vi "Begin.vi"(11 "Image Size":T1=enum."160x120") -> (0 "error out":errorcluster)   [LabVIEW 2012]
doc: "Called before other user functions, this VI is expected to open initial I/O refnums, load in file data, and do all program initialization. Notice that the <B>error out</B> terminal is simply used for data flow. Wiring it to other structures or subVIs ensures that this VI runs first."
uses:
  <vilib>/Rock Robotics/WPI/Camera/WPI_CameraImageSize.ctl
  <vilib>/Rock Robotics/WPI/Camera/WPI_CameraWhite Balance Values.ctl
  <vilib>/Rock Robotics/WPI/Camera/WPI_CameraExposure Values.ctl
  <vilib>/Rock Robotics/WPI/Camera/WPI_CameraFrameRate.ctl
  <vilib>/Rock Robotics/SystemInterfaces/DIO/FPGA_DIOPWMChannel.ctl
  <vilib>/Rock Robotics/SystemInterfaces/Typedef/FPGA_TypedefDigitalModule.ctl
  <vilib>/Rock Robotics/SystemInterfaces/DIO/FPGA_DIOChannel.ctl
  <vilib>/Rock Robotics/WPI/Encoder/WPI_EncoderType.ctl
  <vilib>/Rock Robotics/SystemInterfaces/Typedef/FPGA_TypedefAnalogModuleForGyro.ctl
  <vilib>/Rock Robotics/SystemInterfaces/AI/FPGA_AIGyroChannel.ctl
  <vilib>/Rock Robotics/WPI/SafetyOutput/WPI_SafetyOutputConfigMenu.ctl
  <vilib>/Rock Robotics/WPI/Joystick/WPI_JoystickDeviceEnum.ctl
  <vilib>/Rock Robotics/SystemInterfaces/DIO/FPGA_DIORelayChannel.ctl
  <vilib>/Rock Robotics/SystemInterfaces/Typedef/FPGA_TypedefSolenoidModule.ctl
  <vilib>/Rock Robotics/WPI/Solenoid/WPI_SolenoidChannel.ctl
  <vilib>/Rock Robotics/WPI/MotorControl/WPI_MotorControlOpen Victor.vi
  <vilib>/Rock Robotics/WPI/Counter/WPI_CounterDigitalInputToDigitalSource.vi
  <vilib>/Rock Robotics/WPI/RobotDrive/WPI_RobotDriveOpen4MotorWithVictor.vi
  System Set Points and States.vi
  <vilib>/Rock Robotics/WPI/Counter/WPI_CounterOpen UpDown Mode.vi
  <vilib>/Rock Robotics/WPI/Solenoid/WPI_SolenoidOpenSingle.vi
  <vilib>/Rock Robotics/WPI/Compressor/WPI_CompressorGetSetRefNum.vi
panel:
  in  "Image Size 2":T1=enum."160x120"
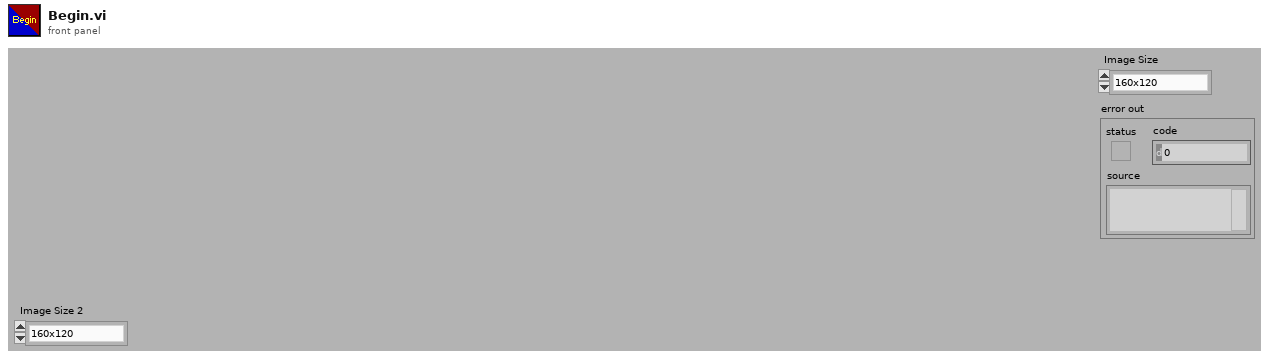
[diagram p1: front panel]
types:
  T1 = typedef "WPI_CameraImageSize.ctl" = enum16{"640x480", "320x240", "160x120"}
  T2 = typedef "WPI_SolenoidChannel.ctl" = enum8{"Solenoid 1", "Solenoid 2", "Solenoid 3", "Solenoid 4", "Solenoid 5", "Solenoid 6", "Solenoid 7", "Solenoid 8", "Invalid"}
  T3 = typedef "FPGA_TypedefSolenoidModule.ctl" = enum16{"Solenoid Module 1", "Solenoid Module 2"}
  T4 = typedef "FPGA_DIORelayChannel.ctl" = enum8{"Relay 1", "Relay 2", "Relay 3", "Relay 4", "Relay 5", "Relay 6", "Relay 7", "Relay 8", "Invalid"}
  T5 = typedef "FPGA_TypedefDigitalModule.ctl" = enum16{"Digital Module 1", "Digital Module 2"}
  T6 = typedef "FPGA_DIOChannel.ctl" = enum8{"DIO 1", "DIO 2", "DIO 3", "DIO 4", "DIO 5", "DIO 6", "DIO 7", "DIO 8", "DIO 9", "DIO 10", "DIO 11", "DIO 12", "DIO 13", "DIO 14", "Invalid"}
  T7 = typedef "WPI_EncoderType.ctl" = enum16{"1x", "2x", "4x"}
  T8 = typedef "WPI_JoystickDeviceEnum.ctl" = enum16{"USB 1", "USB 2", "USB 3", "USB 4", "Kinect 1", "Kinect 2"}
  T9 = typedef "WPI_CameraFrameRate.ctl" = u32
  T10 = typedef "WPI_CameraExposure Values.ctl" = enum16{"Auto", "Flicker-free 50 Hz", "Flicker-free 60 Hz", "Hold current"}
  T11 = typedef "WPI_CameraWhite Balance Values.ctl" = enum16{"Auto", "Fixed indoor", "Fixed outdoor 1", "Fixed outdoor 2", "Fixed fluorescent 1", "Fixed fluorescent 2", "Hold current"}
  T12 = typedef "WPI_SafetyOutputConfigMenu.ctl" = enum16{"Enable", "Disable"}
  T13 = typedef "FPGA_AIGyroChannel.ctl" = enum8{"AI 1", "AI 2", "Invalid"}
  T14 = typedef "FPGA_TypedefAnalogModuleForGyro.ctl" = enum16{"Analog Module 1"}
  T15 = typedef "FPGA_DIOPWMChannel.ctl" = enum8{"PWM 1", "PWM 2", "PWM 3", "PWM 4", "PWM 5", "PWM 6", "PWM 7", "PWM 8", "PWM 9", "PWM 10", "Invalid"}
  T16 = typedef "WPI_RobotDriveDevRef.ctl" = cluster{"DevStatus":errorcluster, "Motors[]":T17[], "Square Inputs":bool, "Max Output":dbl, "Isochronous":bool}
  T17 = typedef "WPI_MotorControlDeviceRef.ctl" = cluster{"DeviceStatus":errorcluster, "Type":enum16{"PWM", "CAN"}, "PWM":cluster{"Digital Module":T5, "PWM Channel":T15, "DeadBand":T18}, "CAN":cluster{"Device Number":u8, "Control Mode":T19, "Semaphore":T20, "Max Vout":dbl}, "Invert":bool, "TransformRef":T21, "InvTransformRef":T21}
  T18 = typedef "WPI_PWMDeadband.ctl" = cluster{"Name":string, "maxPositivePwm":i32, "minPositivePwm":i32, "centerPwm":i32, "maxNegativePwm":i32, "minNegativePwm":i32, "angularRange":u16}
  T19 = typedef "WPI_CANJaguar_ControlMode.ctl" = enum8{"Percent VBus", "Current", "Speed", "Position", "Voltage"}
  T20 = typedef "Semaphore RefNum" = refnum<k1>
  T21 = typedef "WPI_PWMTransform_ConPane.ctl" = refnum<vi>
  T22 = typedef "WPI_CameraDevRef.ctl" = cluster{"Camera Address":string, "CameraStatus":errorcluster, "Acquire Image Notifier":refnum<notifier>}
  T23 = typedef "WPI_DigitalInputDevRef.ctl" = cluster{"DevStatus":errorcluster, "DIO Channel":T6, "Digital Module":T5}
  T24 = typedef "FPGA_CounterEncoderSourceConvertionLVSourceType.ctl" = cluster{"DevStatus":errorcluster, "AnalogTriggerMode?":bool, "DigitalMode":cluster{"Digital Module":T5, "DIO Channel":T25}, "AnalogTriggerMode":cluster{"AnalogTriggerIndex":T26, "OutputType":T27}}
  T25 = typedef "FPGA_DIODigitalSourceChannel.ctl" = enum8{"DIO 1", "DIO 2", "DIO 3", "DIO 4", "DIO 5", "DIO 6", "DIO 7", "DIO 8", "DIO 9", "DIO 10", "DIO 11", "DIO 12", "DIO 13", "DIO 14", "Disabled"}
  T26 = typedef "FPGA_AnalogTriggerIndex.ctl" = enum8{"Trig 0", "Trig 1", "Trig 2", "Trig 3", "Trig 4", "Trig 5", "Trig 6", "Trig 7", "Invalid"}
  T27 = typedef "FPGA_AnalogTriggerOutType.ctl" = enum16{"InWindow", "TriggerState", "Rising", "Falling"}
  T28 = typedef "WPI_GyroDevRef.ctl" = cluster{"DevStatus":errorcluster, "Analog Module":T29, "Analog Channel":T30, "Offset":dbl, "Gain (VoltsPerDegree/Second)":dbl}
  T29 = typedef "FPGA_TypedefAnalogModule.ctl" = enum16{"Analog Module 1", "Analog Module 2"}
  T30 = typedef "FPGA_AIChannel.ctl" = enum8{"AI 1", "AI 2", "AI 3", "AI 4", "AI 5", "AI 6", "AI 7", "AI 8", "Invalid"}
  T31 = typedef "WPI_CounterDevRef.ctl" = cluster{"DevStatus":errorcluster, "CntIndex":T32}
  T32 = typedef "FPGA_CounterCtrSystemIndex.ctl" = enum8{"Ctr 0", "Ctr 1", "Ctr 2", "Ctr 3", "Ctr 4", "Ctr 5", "Ctr 6", "Ctr 7", "Invalid"}
  T33 = typedef "WPI_EncoderDevRef.ctl" = cluster{"DevStatus":errorcluster, "EncoderIndex":T34, "CounterIndex":T32, "DistancePerCount":dbl, "Decoding Type":T7}
  T34 = typedef "FPGA_EncoderIdx.ctl" = enum8{"Enc 0", "Enc 1", "Enc 2", "Enc 3", "Invalid"}
  T35 = typedef "WPI_SolenoidDevRef.ctl" = cluster{"DevStatus":errorcluster, "Solenoid Module":T3, "Forward Solenoid Channel":T2, "Reverse Solenoid Channel":T2}
  T36 = typedef "WPI_CompressorDevRef.ctl" = cluster{"DevStatus":errorcluster, "DigitalInputDevRef":T23, "RelayDevRef":T37}
  T37 = typedef "WPI_RelayDevRef.ctl" = cluster{"DevStatus":errorcluster, "Relay Channel":T4, "Digital Module":T5, "Relay Direction":T38}
  T38 = typedef "WPI_RelayDirection.ctl" = enum16{"Both directions", "Forward only", "Reverse only"}
  T39 = typedef "WPI_JoystickDevRef.ctl" = cluster{"Device":T8}
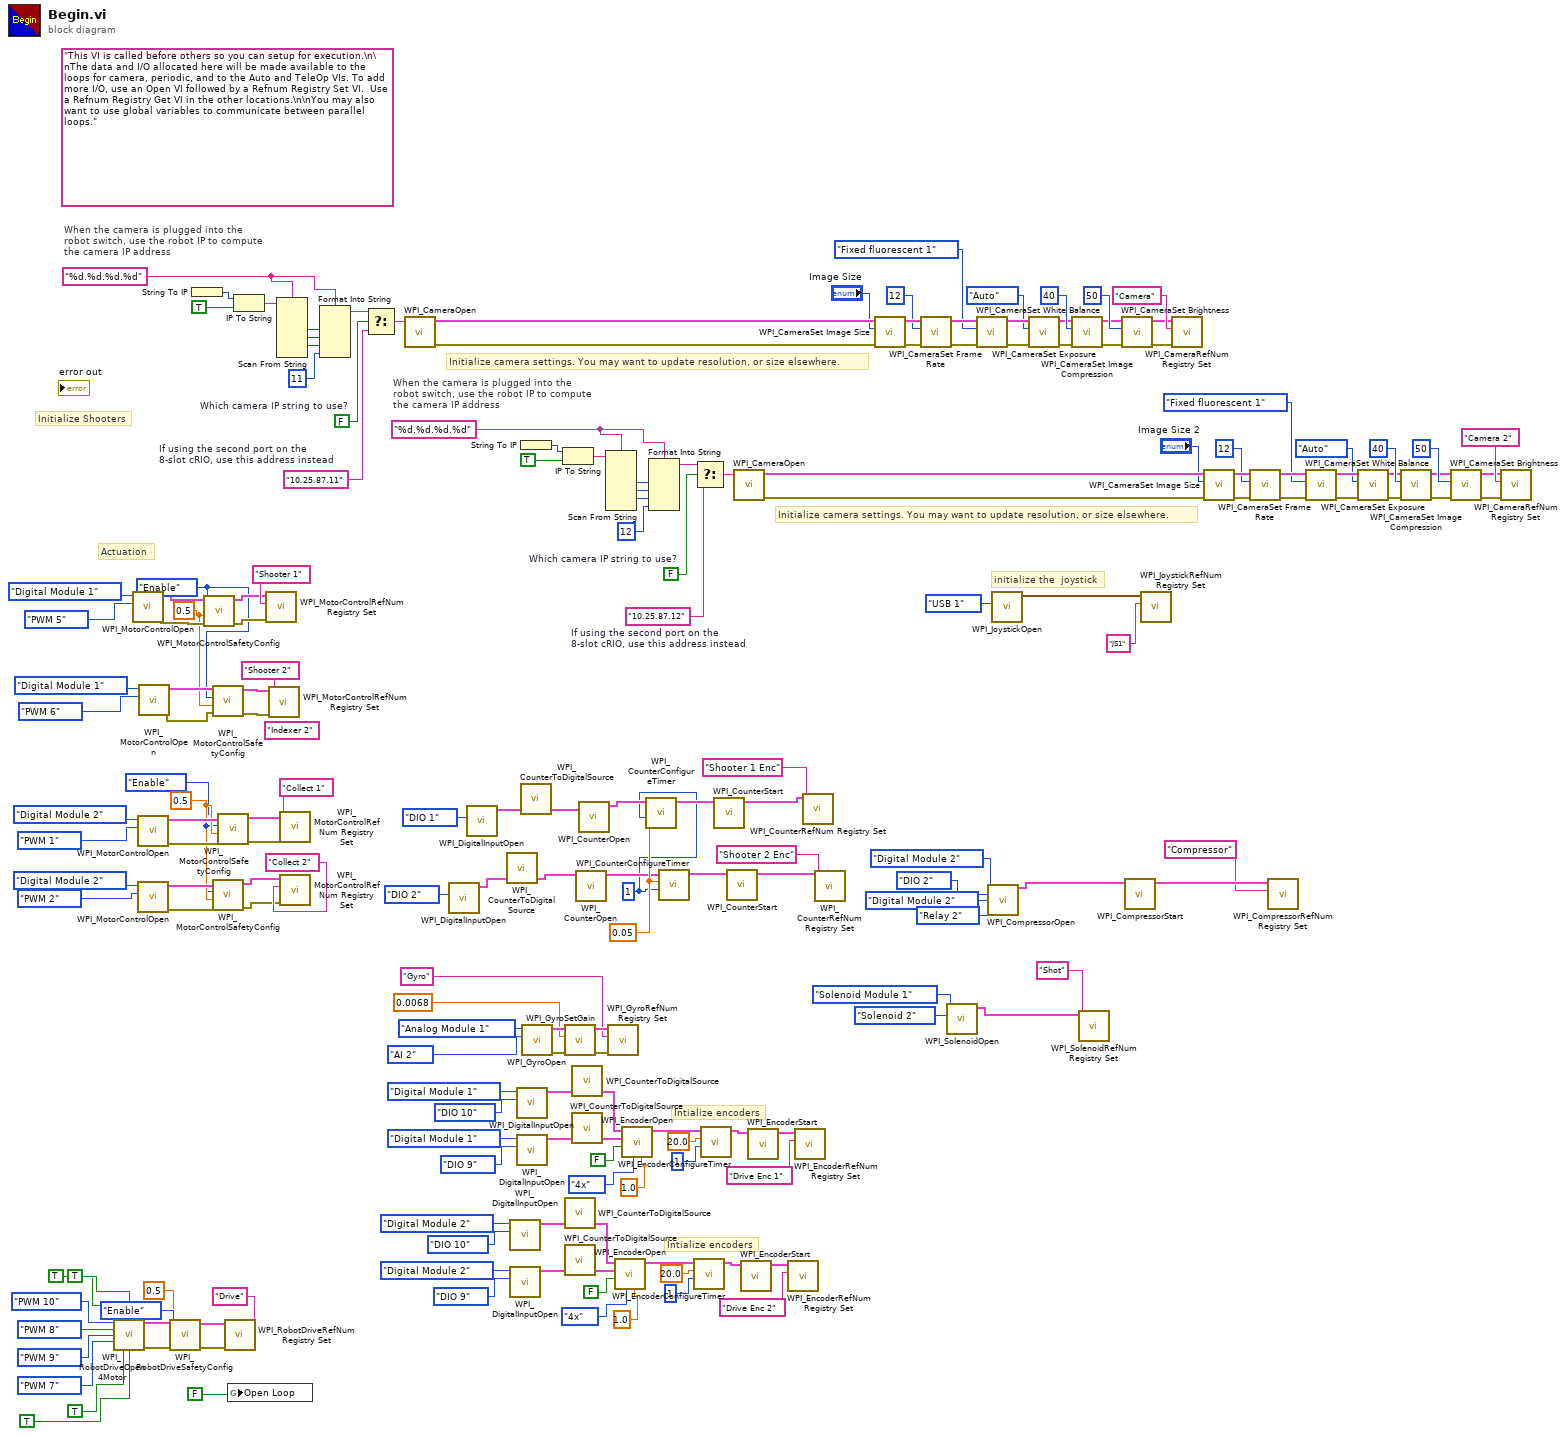
[diagram p0: block diagram]
diagram:
  w12 = u8 1 ("Number Samples to Average")
  w20 = 0.05 ("MaxPeriod (sec)")
  w62 = "10.25.87.12"  # If using the second port on the 8-slot cRIO, use this address instead
  w63 = FALSE  # Which camera IP string to use?
  w66 = "%d.%d.%d.%d" ("format string")
  w31 = WPI_SafetyOutputConfigMenu."Enable" ("mode")
  w22 = WPI_SafetyOutputConfigMenu."Enable" ("mode")
  w32 = 0.5 ("timeout (s)")
  w23 = 0.5 ("timeout (s)")
  (unwired) "Indexer 2" ("refnum name")
  w154 = FALSE  # Which camera IP string to use?
  w158 = "%d.%d.%d.%d" ("format string")
  (unwired) "This VI is called before others so you can setup for execution.\n\nThe data and I/O allocated here will be made available to the loops for camera, periodic, and to the Auto and TeleOp VIs. To add more I/O, use an Open VI followed by a Refnum Registry Set VI.  Use a Refnum Registry Get VI in the other locations.\n\nYou may also want to use global variables to communicate between parallel loops."
  w155 = "10.25.87.11"  # If using the second port on the 8-slot cRIO, use this address instead
  # "Intialize encoders"
  # "initialize the  joystick"
  # "When the camera is plugged into the\nrobot switch, use the robot IP to compute\nthe camera IP address"
  # "Initialize camera settings. You may want to update resolution, or size elsewhere."
  # "Intialize encoders"
  # "Actuation"
  # "Initialize Shooters"
  # "When the camera is plugged into the\nrobot switch, use the robot IP to compute\nthe camera IP address"
  # "Initialize camera settings. You may want to update resolution, or size elsewhere."
  n1 = call-poly <vilib>:"WPI_RobotDriveOpen4Motor.vi"("Rear Left Motor"=FPGA_DIOPWMChannel."PWM 10", "Rear Left Motor Inverted"=TRUE, "Rear Right Motor Inverted"=TRUE, "Rear Right Motor"=FPGA_DIOPWMChannel."PWM 8", "Front Left Motor"=FPGA_DIOPWMChannel."PWM 9", "Front Right Motor"=FPGA_DIOPWMChannel."PWM 7", "Front Left Motor Inverted"=TRUE, "Front Right Motor Inverted"=TRUE) -> ("RobotDriveDevRef"=w98:T16, "error out"=w99:errorcluster)  [unwired: 6 in]
  n2 = call-poly <vilib>:"WPI_MotorControlOpen.vi"("PWM Channel"=FPGA_DIOPWMChannel."PWM 5", "Digital Module (Module 1)"=FPGA_TypedefDigitalModule."Digital Module 1") -> ("error out"=w105:errorcluster, "MotorControlDeviceRef"=w107:T17)  [unwired: 8 in]
  n3 = call-poly <vilib>:"WPI_MotorControlOpen.vi"("PWM Channel"=FPGA_DIOPWMChannel."PWM 1", "Digital Module (Module 1)"=FPGA_TypedefDigitalModule."Digital Module 2") -> ("error out"=w59:errorcluster, "MotorControlDeviceRef"=w61:T17)  [unwired: 8 in]
  n4 = call-poly <vilib>:"WPI_MotorControlOpen.vi"("PWM Channel"=FPGA_DIOPWMChannel."PWM 2", "Digital Module (Module 1)"=FPGA_TypedefDigitalModule."Digital Module 2") -> ("error out"=w55:errorcluster, "MotorControlDeviceRef"=w57:T17)  [unwired: 8 in]
  n5 = call-poly <vilib>:"WPI_MotorControlOpen.vi"("PWM Channel"=FPGA_DIOPWMChannel."PWM 6", "Digital Module (Module 1)"=FPGA_TypedefDigitalModule."Digital Module 1") -> ("error out"=w100:errorcluster, "MotorControlDeviceRef"=w101:T17)  [unwired: 8 in]
  n6 = call <vilib>:"WPI_RobotDriveSafetyConfig.vi"("error in (no error)"=w99, "timeout (s)"=0.5, "mode"=WPI_SafetyOutputConfigMenu."Enable", "RobotDriveDevRef"=w98) -> ("error out"=w96:errorcluster, "RobotDriveDevRef"=w97:T16)  [unwired: 6 in]
  n7 = String To IP() -> (0:w165:u32)  [unwired: 1 in]
  n8 = call <vilib>:"WPI_MotorControlSafetyConfig.vi"("error in (no error)"=w105, "timeout (s)"=w23, "mode"=w22, "MotorControlDevRef"=w107) -> ("error out"=w104:errorcluster, "MotorControlDevRef"=w106:T17)  [unwired: 6 in]
  n9 = call <vilib>:"WPI_MotorControlSafetyConfig.vi"("error in (no error)"=w100, "timeout (s)"=w23, "mode"=w22, "MotorControlDevRef"=w101) -> ("error out"=w103:errorcluster, "MotorControlDevRef"=w102:T17)  [unwired: 6 in]
  n10 = call <vilib>:"WPI_MotorControlSafetyConfig.vi"("error in (no error)"=w55, "timeout (s)"=w32, "mode"=w31, "MotorControlDevRef"=w57) -> ("error out"=w54:errorcluster, "MotorControlDevRef"=w56:T17)  [unwired: 6 in]
  n11 = call <vilib>:"WPI_MotorControlSafetyConfig.vi"("error in (no error)"=w59, "timeout (s)"=w32, "mode"=w31, "MotorControlDevRef"=w61) -> ("error out"=w58:errorcluster, "MotorControlDevRef"=w60:T17)  [unwired: 6 in]
  n12 = call <vilib>:"WPI_RobotDriveRefNum Registry Set.vi"("error in (no error)"=w96, "refnum name"="Drive", "RobotDriveDevRef"=w97) -> ()  [unwired: 7 in, 2 out]
  n13 = global write "System Set Points and States.vi" "Open Loop"(FALSE) -> ()
  n14 = IP To String(1:TRUE ("dot notation? (F)"), 2:w165) -> (0:w163:string)
  n15 = call <vilib>:"WPI_MotorControlRefNum Registry Set.vi"("error in (no error)"=w104, "refnum name"="Shooter 1", "MotorControlDevRef"=w106) -> ()  [unwired: 7 in, 2 out]
  n16 = call <vilib>:"WPI_MotorControlRefNum Registry Set.vi"("error in (no error)"=w103, "refnum name"="Shooter 2", "MotorControlDevRef"=w102) -> ()  [unwired: 7 in, 2 out]
  n17 = Scan From String(format string=w158, input string=w163) -> (output 1=w162:i32, output 2=w161:i32, output 3=w160:i32)  [unwired: 7 in, 3 out]
  n18 = call <vilib>:"WPI_MotorControlRefNum Registry Set.vi"("error in (no error)"=w58, "refnum name"="Collect 1", "MotorControlDevRef"=w60) -> ()  [unwired: 7 in, 2 out]
  n19 = call <vilib>:"WPI_MotorControlRefNum Registry Set.vi"("error in (no error)"=w54, "refnum name"="Collect 2", "MotorControlDevRef"=w56) -> ()  [unwired: 7 in, 2 out]
  n20 = Format Into String(format string=w158, w162, w161, w160, 11 ("Compression")) -> (resulting string=w156:string)  [unwired: 2 in, 1 out]
  n21 = Select(t=w156, s=w154, f=w155) -> (s? t:f=w157:string)
  n22 = call <vilib>:"WPI_CameraOpen.vi"("Camera Address"=w157) -> ("error out"=w177:errorcluster, "CameraDevRef"=w178:T22)  [unwired: 1 in, 8 out]
  n23 = call <vilib>:"WPI_DigitalInputOpen.vi"("DIO Channel"=FPGA_DIOChannel."DIO 2") -> ("DigitalInputDevRef"=w25:T23)  [unwired: 9 in, 1 out]
  n24 = call <vilib>:"WPI_DigitalInputOpen.vi"("DIO Channel"=FPGA_DIOChannel."DIO 1") -> ("DigitalInputDevRef"=w28:T23)  [unwired: 9 in, 1 out]
  n25 = call-poly <vilib>:"WPI_CounterToDigitalSource.vi"("DigitalInputDevRef"=w25) -> ("Digital Source"=w26:T24)  [unwired: 6 in]
  n26 = call <vilib>:"WPI_DigitalInputOpen.vi"("DIO Channel"=FPGA_DIOChannel."DIO 10", "Digital Module (Module 1)"=FPGA_TypedefDigitalModule."Digital Module 2") -> ("DigitalInputDevRef"=w47:T23)  [unwired: 8 in, 1 out]
  n27 = call <vilib>:"WPI_DigitalInputOpen.vi"("DIO Channel"=FPGA_DIOChannel."DIO 9", "Digital Module (Module 1)"=FPGA_TypedefDigitalModule."Digital Module 2") -> ("DigitalInputDevRef"=w43:T23)  [unwired: 8 in, 1 out]
  n28 = call <vilib>:"WPI_DigitalInputOpen.vi"("DIO Channel"=FPGA_DIOChannel."DIO 10", "Digital Module (Module 1)"=FPGA_TypedefDigitalModule."Digital Module 1") -> ("DigitalInputDevRef"=w142:T23)  [unwired: 8 in, 1 out]
  n29 = call <vilib>:"WPI_DigitalInputOpen.vi"("DIO Channel"=FPGA_DIOChannel."DIO 9", "Digital Module (Module 1)"=FPGA_TypedefDigitalModule."Digital Module 1") -> ("DigitalInputDevRef"=w138:T23)  [unwired: 8 in, 1 out]
  n30 = String To IP() -> (0:w73:u32)  [unwired: 1 in]
  n31 = call-poly <vilib>:"WPI_CounterToDigitalSource.vi"("DigitalInputDevRef"=w28) -> ("Digital Source"=w29:T24)  [unwired: 6 in]
  n32 = call <vilib>:"WPI_GyroOpen.vi"("Analog Channel"=FPGA_AIGyroChannel."AI 2", "Analog Module (Module 1)"=FPGA_TypedefAnalogModuleForGyro."Analog Module 1") -> ("error out"=w118:errorcluster, "GyroDevRef"=w117:T28)  [unwired: 7 in, 1 out]
  n33 = IP To String(1:TRUE ("dot notation? (F)"), 2:w73) -> (0:w71:string)
  n34 = call <vilib>:"WPI_GyroSetGain.vi"("error in (no error)"=w118, "Gain (VoltsPerDegree/Second)"=0.0068, "GyroDevRef"=w117) -> ("error out"=w114:errorcluster, "GyroDevRef"=w116:T28)  [unwired: 7 in]
  n35 = call-poly <vilib>:"WPI_CounterToDigitalSource.vi"("DigitalInputDevRef"=w47) -> ("Digital Source"=w46:T24)  [unwired: 6 in]
  n36 = call-poly <vilib>:"WPI_CounterToDigitalSource.vi"("DigitalInputDevRef"=w43) -> ("Digital Source"=w42:T24)  [unwired: 6 in]
  n37 = call-poly <vilib>:"WPI_CounterToDigitalSource.vi"("DigitalInputDevRef"=w142) -> ("Digital Source"=w141:T24)  [unwired: 6 in]
  n38 = call-poly <vilib>:"WPI_CounterToDigitalSource.vi"("DigitalInputDevRef"=w138) -> ("Digital Source"=w137:T24)  [unwired: 6 in]
  n39 = call-poly <vilib>:"WPI_CounterOpen.vi"("Up Source"=w26) -> ("CounterDevRef"=w19:T31)  [unwired: 9 in, 1 out]
  n40 = call-poly <vilib>:"WPI_CounterOpen.vi"("Up Source"=w29) -> ("CounterDevRef"=w21:T31)  [unwired: 9 in, 1 out]
  n41 = Scan From String(format string=w66, input string=w71) -> (output 1=w70:i32, output 2=w69:i32, output 3=w68:i32)  [unwired: 7 in, 3 out]
  n42 = call <vilib>:"WPI_GyroRefNum Registry Set.vi"("error in (no error)"=w114, "refnum name"="Gyro", "GyroDevRef"=w116) -> ()  [unwired: 7 in, 2 out]
  n43 = call <vilib>:"WPI_EncoderOpen.vi"("DistancePerCount"=1.0, "Decoding Type"=WPI_EncoderType."4x", "Invert Direction (False)"=FALSE, "BSource"=w42, "ASource"=w46) -> ("EncoderDevRef"=w40:T33)  [unwired: 5 in, 1 out]
  n44 = call <vilib>:"WPI_EncoderOpen.vi"("DistancePerCount"=1.0, "Decoding Type"=WPI_EncoderType."4x", "Invert Direction (False)"=FALSE, "BSource"=w137, "ASource"=w141) -> ("EncoderDevRef"=w135:T33)  [unwired: 5 in, 1 out]
  n45 = call <vilib>:"WPI_CounterConfigureTimer.vi"("Number Samples to Average"=w12, "MaxPeriod (sec)"=w20, "CounterDevRef in"=w21) -> ("CounterDevRef out"=w18:T31)  [unwired: 7 in, 1 out]
  n46 = Format Into String(format string=w66, w70, w69, w68, 12 ("Compression")) -> (resulting string=w64:string)  [unwired: 2 in, 1 out]
  n47 = call <vilib>:"WPI_CounterConfigureTimer.vi"("Number Samples to Average"=w12, "MaxPeriod (sec)"=w20, "CounterDevRef in"=w19) -> ("CounterDevRef out"=w17:T31)  [unwired: 7 in, 1 out]
  n48 = call <vilib>:"WPI_EncoderConfigureTimer.vi"("Number Samples to Average"=u8 1, "Minimum Rate"=20.0, "EncoderDevRef"=w40) -> ("EncoderDevRef"=w34:T33)  [unwired: 7 in, 1 out]
  n49 = Select(t=w64, s=w63, f=w62) -> (s? t:f=w65:string)
  n50 = call <vilib>:"WPI_EncoderConfigureTimer.vi"("Number Samples to Average"=u8 1, "Minimum Rate"=20.0, "EncoderDevRef"=w135) -> ("EncoderDevRef"=w110:T33)  [unwired: 7 in, 1 out]
  n51 = call <vilib>:"WPI_CounterStart.vi"("CounterDevRef in"=w18) -> ("CounterDevRef out"=w16:T31)  [unwired: 9 in, 1 out]
  n52 = call <vilib>:"WPI_CounterStart.vi"("CounterDevRef in"=w17) -> ("CounterDevRef out"=w15:T31)  [unwired: 9 in, 1 out]
  n53 = call <vilib>:"WPI_CameraOpen.vi"("Camera Address"=w65) -> ("error out"=w84:errorcluster, "CameraDevRef"=w85:T22)  [unwired: 1 in, 8 out]
  n54 = call <vilib>:"WPI_EncoderStart.vi"("EncoderDevRef"=w34) -> ("EncoderDevRef"=w33:T33)  [unwired: 9 in, 1 out]
  n55 = call <vilib>:"WPI_EncoderStart.vi"("EncoderDevRef"=w110) -> ("EncoderDevRef"=w109:T33)  [unwired: 9 in, 1 out]
  n56 = call <vilib>:"WPI_EncoderRefNum Registry Set.vi"("refnum name"="Drive Enc 2", "EncoderDevRef"=w33) -> ()  [unwired: 8 in, 2 out]
  n57 = call <vilib>:"WPI_EncoderRefNum Registry Set.vi"("refnum name"="Drive Enc 1", "EncoderDevRef"=w109) -> ()  [unwired: 8 in, 2 out]
  n58 = call <vilib>:"WPI_CounterRefNum Registry Set.vi"("refnum name"="Shooter 1 Enc", "CounterDevRef"=w16) -> ()  [unwired: 8 in, 2 out]
  n59 = call <vilib>:"WPI_CounterRefNum Registry Set.vi"("refnum name"="Shooter 2 Enc", "CounterDevRef"=w15) -> ()  [unwired: 8 in, 2 out]
  n60 = call <vilib>:"WPI_CameraSet Image Size.vi"("error in (no error)"=w177, "Image Size"="Image Size", "CameraDevRef"=w178) -> ("error out"=w176:errorcluster, "CameraDevRef Out"=w179:T22)  [unwired: 7 out]
  n61 = call <vilib>:"WPI_CameraSet Frame Rate.vi"("error in (no error)"=w176, "Frame Rate (fps)"=T9 12, "CameraDevRef"=w179) -> ("error out"=w175:errorcluster, "CameraDevRef Out"=w181:T22)  [unwired: 7 out]
  n62 = call-poly <vilib>:"WPI_SolenoidOpen.vi"("Solenoid Channel"=WPI_SolenoidChannel."Solenoid 2", "Solenoid Module (Module 1)"=FPGA_TypedefSolenoidModule."Solenoid Module 1") -> ("SolenoidDevRef"=w2:T35)  [unwired: 8 in, 1 out]
  n63 = call <vilib>:"WPI_CameraSet White Balance.vi"("error in (no error)"=w175, "White Balance"=WPI_CameraWhite_Balance_Values."Fixed fluorescent 1", "CameraDevRef"=w181) -> ("error out"=w174:errorcluster, "CameraDevRef Out"=w180:T22)  [unwired: 7 out]
  n64 = call <vilib>:"WPI_CompressorOpen.vi"("Pressure Switch Digital Module (Module 1)"=FPGA_TypedefDigitalModule."Digital Module 2", "Pressure Switch DIO Channel"=FPGA_DIOChannel."DIO 2", "Relay Digital Module (Module 1)"=FPGA_TypedefDigitalModule."Digital Module 2", "Relay Channel"=FPGA_DIORelayChannel."Relay 2") -> ("CompressorDevRef"=w9:T36)  [unwired: 10 in, 1 out]
  n65 = call <vilib>:"WPI_JoystickOpen.vi"("JoystickDevice"=WPI_JoystickDeviceEnum."USB 1") -> ("JoystickDevRef"=w51:T39)  [unwired: 10 out]
  n66 = call <vilib>:"WPI_CameraSet Exposure.vi"("error in (no error)"=w174, "Exposure"=WPI_CameraExposure_Values."Auto", "CameraDevRef"=w180) -> ("error out"=w173:errorcluster, "CameraDevRef Out"=w183:T22)  [unwired: 7 out]
  n67 = call <vilib>:"WPI_CameraSet Image Compression.vi"("error in (no error)"=w173, "Compression"=40, "CameraDevRef"=w183) -> ("error out"=w172:errorcluster, "CameraDevRef Out"=w182:T22)  [unwired: 7 out]
  n68 = call <vilib>:"WPI_SolenoidRefNum Registry Set.vi"("refnum name"="Shot", "SolenoidDevRef"=w2) -> ()  [unwired: 8 in, 2 out]
  n69 = call <vilib>:"WPI_CameraSet Brightness.vi"("error in (no error)"=w172, "Brightness"=50, "CameraDevRef"=w182) -> ("error out"=w170:errorcluster, "CameraDevRef Out"=w171:T22)  [unwired: 7 out]
  n70 = call <vilib>:"WPI_CompressorStart.vi"("CompressorDevRef"=w9) -> ("CompressorDevRef"=w11:T36)  [unwired: 9 in, 1 out]
  n71 = call <vilib>:"WPI_JoystickRefNum Registry Set.vi"("refnum name"="JS1", "JoystickDevRef"=w51) -> ()  [unwired: 1 in, 9 out]
  n72 = call <vilib>:"WPI_CameraRefNum Registry Set.vi"("error in (no error)"=w170, "refnum name"="Camera", "CameraDevRef"=w171) -> ()  [unwired: 9 out]
  n73 = call <vilib>:"WPI_CameraSet Image Size.vi"("error in (no error)"=w84, "Image Size"="Image Size 2", "CameraDevRef"=w85) -> ("error out"=w83:errorcluster, "CameraDevRef Out"=w86:T22)  [unwired: 7 out]
  n74 = call <vilib>:"WPI_CameraSet Frame Rate.vi"("error in (no error)"=w83, "Frame Rate (fps)"=T9 12, "CameraDevRef"=w86) -> ("error out"=w82:errorcluster, "CameraDevRef Out"=w88:T22)  [unwired: 7 out]
  n75 = call <vilib>:"WPI_CompressorRefNum Registry Set.vi"("refnum name"="Compressor", "CompressorDevRef"=w11) -> ()  [unwired: 8 in, 2 out]
  n76 = call <vilib>:"WPI_CameraSet White Balance.vi"("error in (no error)"=w82, "White Balance"=WPI_CameraWhite_Balance_Values."Fixed fluorescent 1", "CameraDevRef"=w88) -> ("error out"=w81:errorcluster, "CameraDevRef Out"=w87:T22)  [unwired: 7 out]
  n77 = call <vilib>:"WPI_CameraSet Exposure.vi"("error in (no error)"=w81, "Exposure"=WPI_CameraExposure_Values."Auto", "CameraDevRef"=w87) -> ("error out"=w80:errorcluster, "CameraDevRef Out"=w90:T22)  [unwired: 7 out]
  n78 = call <vilib>:"WPI_CameraSet Image Compression.vi"("error in (no error)"=w80, "Compression"=40, "CameraDevRef"=w90) -> ("error out"=w79:errorcluster, "CameraDevRef Out"=w89:T22)  [unwired: 7 out]
  n79 = call <vilib>:"WPI_CameraSet Brightness.vi"("error in (no error)"=w79, "Brightness"=50, "CameraDevRef"=w89) -> ("error out"=w77:errorcluster, "CameraDevRef Out"=w78:T22)  [unwired: 7 out]
  n80 = call <vilib>:"WPI_CameraRefNum Registry Set.vi"("error in (no error)"=w77, "refnum name"="Camera 2", "CameraDevRef"=w78) -> ()  [unwired: 9 out]
